vi "SS_FPGA_Drop1.vi"() -> ()   [LabVIEW 2016]
uses:
  <vilib>/rvi/Emulation/niFpgaGetClockAttributes.vi
  <vilib>/rvi/Emulation/niFpgaSctlEmulationGetInTimedLoop.vi
  <vilib>/rvi/Emulation/niFpgaEmulationReportErrorSimple.vi
  <vilib>/rvi/Emulation/niFpgaCriticalErrorInLSC.vi
  <vilib>/rvi/Emulation/niFpgaProcessEmulError.vi
  <vilib>/rvi/eio/common/nirviEmuTemplateMethod_errors.vi
  <vilib>/eio/EIONode/EIONode.xnode
panel:
  in  "Set Pump Interlock":bool
  out "Raw Data out Mod 3":fxp<+/-,24,-4>[](array[numeric]) format="%.27g"
  out "Raw Data out Mod 2":fxp<+/-,24,-4>[](array[numeric]) format="%.27g"
  in  "Scan Rate (mSec) Loop 1":u32 caption="Count(mSec)"
  out "Raw Data out Mod 1":fxp<+/-,24,-4>[](array[numeric]) format="%.27g"
  out "Number of Loop 1 Samples":i32
  out "Actual Duration (ms)":u32
  in  "Set Flow Interlock":bool
  in  "Start Acquisition":bool
  # "SS Source Body Flow\n\nSS Source Body Temperature\n\nSS Grid 1 Flow\n\nSS Grid 1 Temperature\n\nSS Grid 2 Flow\n\nSS Grid 2 Temperature\n\nSS Grid 3 Flow\n\nSS Grid 3 Temperature\n\nSS Grid 4/1st Stage Neutraliser Flow\n\nSS Grid 4/1st Stage Neutraliser Temperature\n\nSS 2nd Stage Neutraliser Flow\n\nSS 2nd Stage Neutraliser Temperature\n\nSS PINI Backplate Flow\n\nSS PINI Backplate Temperature\n\nSS Duct Scraper Flow\n\nSS Duct Scraper Temperature"
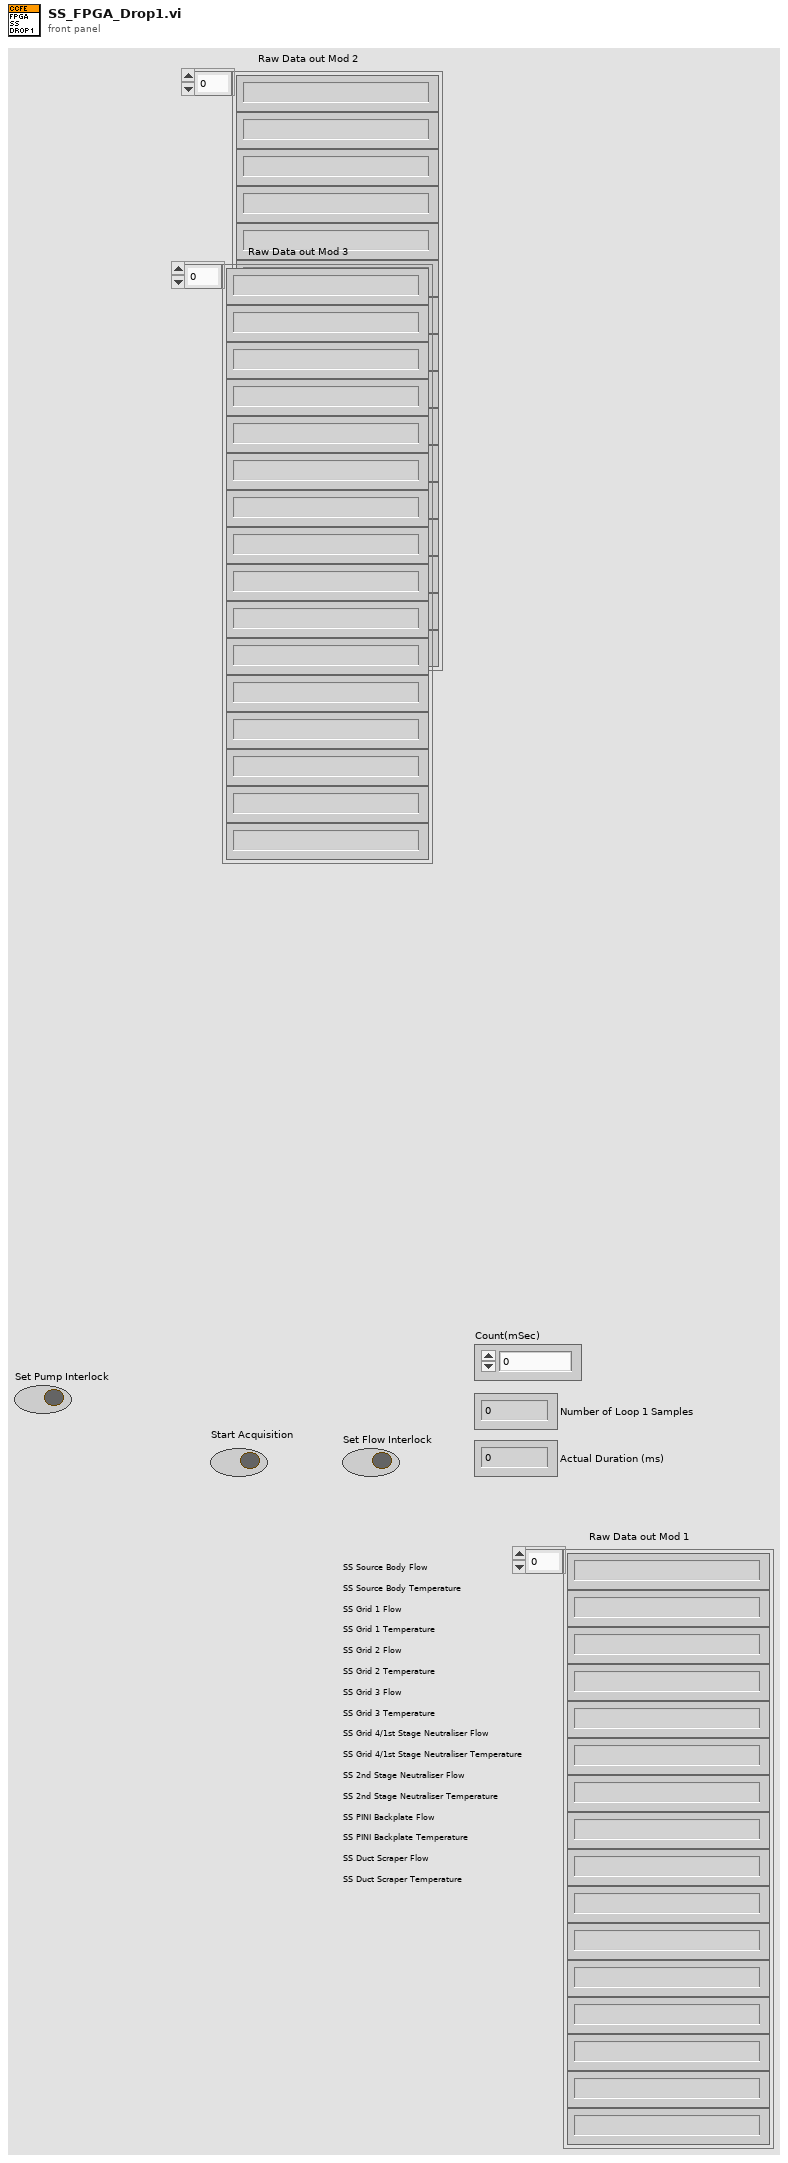
[diagram p1: front panel]
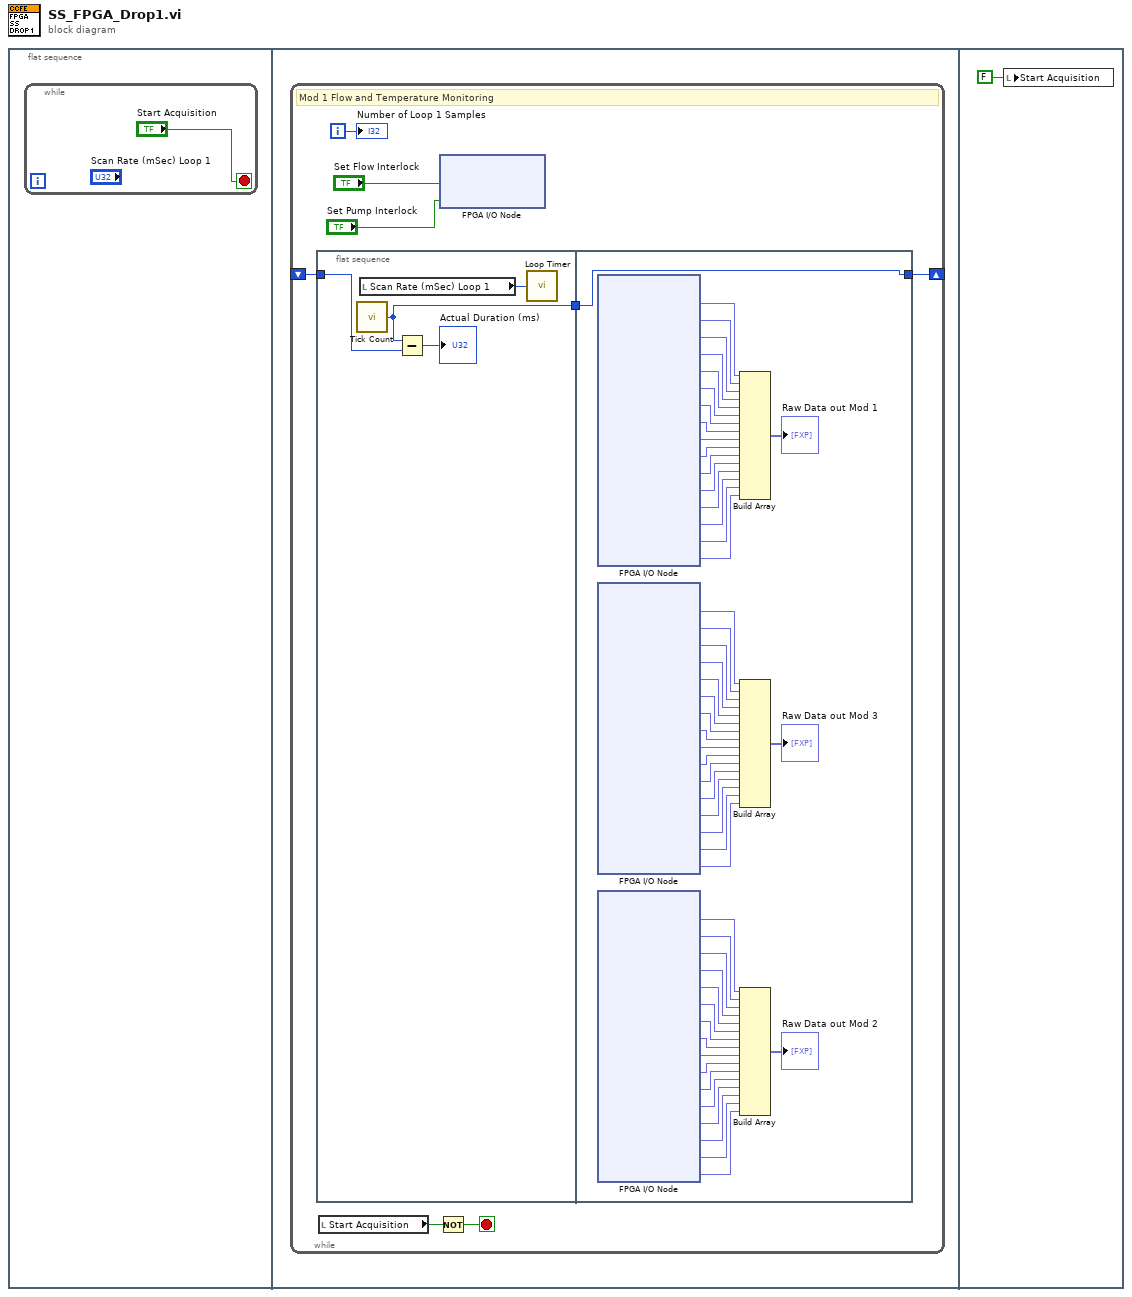
[diagram p0: block diagram]
diagram:
  n1 = flat-sequence {
    frame #0 {
      n2 = while {
        stop <- "Start Acquisition" stop-if-true
      }
    }
    frame #1 {
      n3 = while {
        shift-right: [w8] -> _
        shift-left: _ -> [w6]
        i -> [w9]
        stop <- w5 stop-if-true
        # "Mod 1 Flow and Temperature Monitoring"
        n4 = flat-sequence {
          tunnel: [w10] -> w7
          tunnel: w6 -> [w11]
          tunnel: [w15] -> w8
          tunnel: w7 -> [w15]
          frame #0 {
            n5 = call "Tick Count"() -> ("Tick Count(mSec)"=w10:u32)
            n6 = local read "Scan Rate (mSec) Loop 1"() -> (w13:u32)
            n7 = Subtract(x=w10, y=w11) -> (x-y=→"Actual Duration (ms)":u32)
            n8 = call "Loop Timer"("Count(mSec)"=w13) -> ()  [unwired: 1 out]
          }
          frame #1 {
            n9 = xnode "FPGA I/O Node"() -> ("Mod1/AI0"=w65:fxp<+/-,24,-4>, "Mod1/AI1"=w64:fxp<+/-,24,-4>, "Mod1/AI2"=w63:fxp<+/-,24,-4>, "Mod1/AI3"=w62:fxp<+/-,24,-4>, "Mod1/AI4"=w61:fxp<+/-,24,-4>, "Mod1/AI5"=w60:fxp<+/-,24,-4>, "Mod1/AI6"=w59:fxp<+/-,24,-4>, "Mod1/AI7"=w58:fxp<+/-,24,-4>, "Mod1/AI8"=w57:fxp<+/-,24,-4>, "Mod1/AI9"=w56:fxp<+/-,24,-4>, "Mod1/AI10"=w55:fxp<+/-,24,-4>, "Mod1/AI11"=w54:fxp<+/-,24,-4>, "Mod1/AI12"=w53:fxp<+/-,24,-4>, "Mod1/AI13"=w52:fxp<+/-,24,-4>, "Mod1/AI14"=w51:fxp<+/-,24,-4>, "Mod1/AI15"=w50:fxp<+/-,24,-4>)  [unwired: 16 in, 16 out]
            n10 = xnode "FPGA I/O Node"() -> ("Mod3/AI0"=w32:fxp<+/-,24,-4>, "Mod3/AI1"=w31:fxp<+/-,24,-4>, "Mod3/AI2"=w30:fxp<+/-,24,-4>, "Mod3/AI3"=w29:fxp<+/-,24,-4>, "Mod3/AI4"=w28:fxp<+/-,24,-4>, "Mod3/AI5"=w27:fxp<+/-,24,-4>, "Mod3/AI6"=w26:fxp<+/-,24,-4>, "Mod3/AI7"=w25:fxp<+/-,24,-4>, "Mod3/AI8"=w24:fxp<+/-,24,-4>, "Mod3/AI9"=w23:fxp<+/-,24,-4>, "Mod3/AI10"=w22:fxp<+/-,24,-4>, "Mod3/AI11"=w21:fxp<+/-,24,-4>, "Mod3/AI12"=w20:fxp<+/-,24,-4>, "Mod3/AI13"=w19:fxp<+/-,24,-4>, "Mod3/AI14"=w18:fxp<+/-,24,-4>, "Mod3/AI15"=w17:fxp<+/-,24,-4>)  [unwired: 16 in, 16 out]
            n11 = xnode "FPGA I/O Node"() -> ("Mod2/AI0"=w48:fxp<+/-,24,-4>, "Mod2/AI1"=w47:fxp<+/-,24,-4>, "Mod2/AI2"=w46:fxp<+/-,24,-4>, "Mod2/AI3"=w45:fxp<+/-,24,-4>, "Mod2/AI4"=w44:fxp<+/-,24,-4>, "Mod2/AI5"=w43:fxp<+/-,24,-4>, "Mod2/AI6"=w42:fxp<+/-,24,-4>, "Mod2/AI7"=w41:fxp<+/-,24,-4>, "Mod2/AI8"=w40:fxp<+/-,24,-4>, "Mod2/AI9"=w39:fxp<+/-,24,-4>, "Mod2/AI10"=w38:fxp<+/-,24,-4>, "Mod2/AI11"=w37:fxp<+/-,24,-4>, "Mod2/AI12"=w36:fxp<+/-,24,-4>, "Mod2/AI13"=w35:fxp<+/-,24,-4>, "Mod2/AI14"=w34:fxp<+/-,24,-4>, "Mod2/AI15"=w33:fxp<+/-,24,-4>)  [unwired: 16 in, 16 out]
            n12 = Build Array(w65, w64, w63, w62, w61, w60, w59, w58, w57, w56, w55, w54, w53, w52, w51, w50) -> (→"Raw Data out Mod 1":fxp<+/-,24,-4>[])
            n13 = Build Array(w32, w31, w30, w29, w28, w27, w26, w25, w24, w23, w22, w21, w20, w19, w18, w17) -> (→"Raw Data out Mod 3":fxp<+/-,24,-4>[])
            n14 = Build Array(w48, w47, w46, w45, w44, w43, w42, w41, w40, w39, w38, w37, w36, w35, w34, w33) -> (→"Raw Data out Mod 2":fxp<+/-,24,-4>[])
          }
        }
        n15 = local read "Start Acquisition"() -> (w4:bool)
        n16 = Not(x=w4) -> (.not. x?=w5:bool)
        n17 = xnode "FPGA I/O Node"("Mod6/DIO0"="Set Flow Interlock", "Mod6/DIO1"="Set Pump Interlock") -> ()  [unwired: 2 in, 2 out]
        "Number of Loop 1 Samples" <- w9
      }
    }
    frame #2 {
      n18 = local write "Start Acquisition"(FALSE ("Start Acquisition")) -> ()
    }
  }
